vi "Inject Class Instances.vi"(8 "error in (no error)":errorcluster, 9 "Step in":refnum<class "CallVIStep.lvclass">, 10 "Execution in":refnum<data-value>, 11 "VI Refnum in":refnum<vi>) -> (0 "error out":errorcluster, 3 "VI Refnum out":refnum<vi>)   [LabVIEW 2015, in "CallVIStep.lvclass"]
uses:
  CallVIStep.lvclass
  Execution.lvclass
  Project.lvclass
  <vilib>/Utility/Data Type/NI_Data Type.lvlib
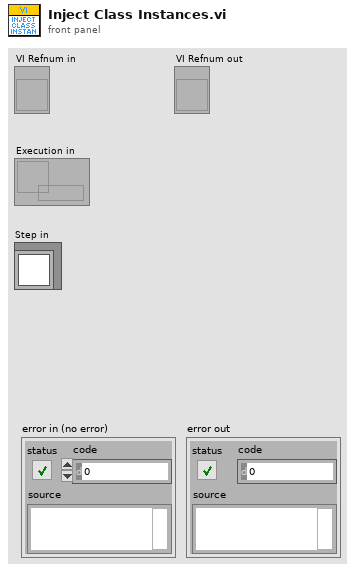
[diagram p1: front panel]
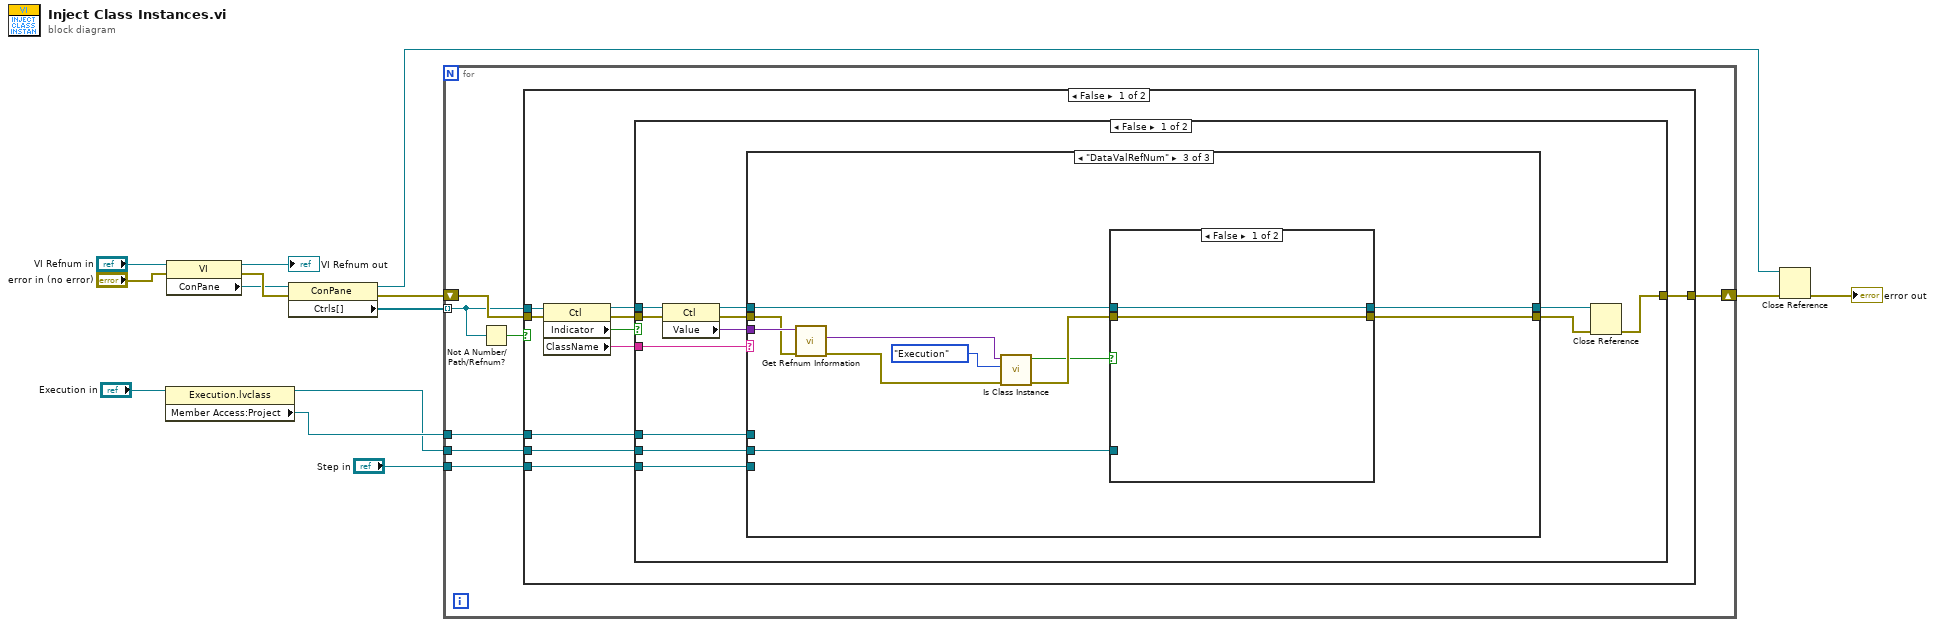
[diagram p0: block diagram]
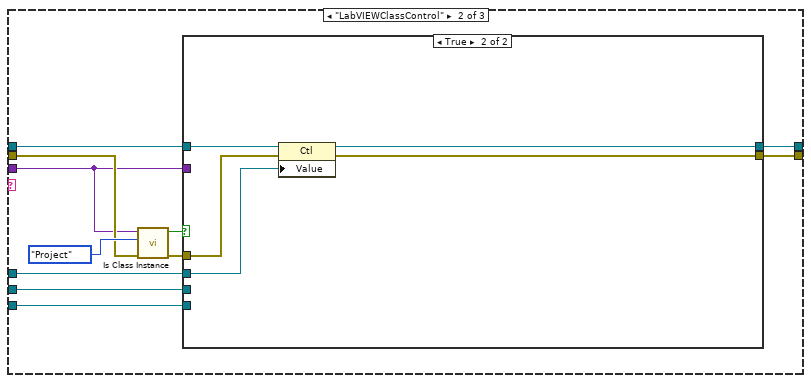
[diagram p3: hidden frame]
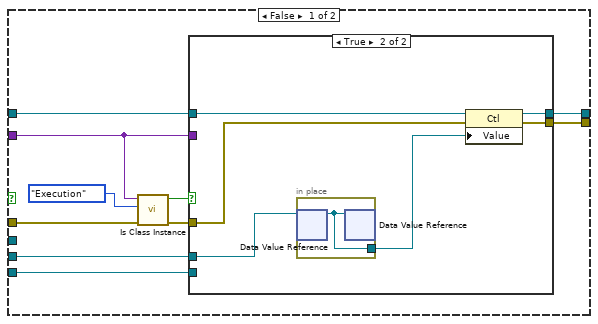
[diagram p4: hidden frame]
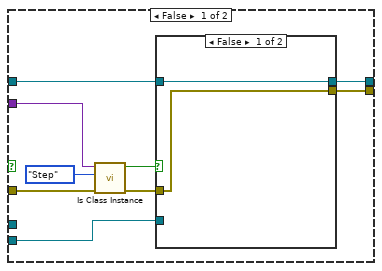
[diagram p5: hidden frame]
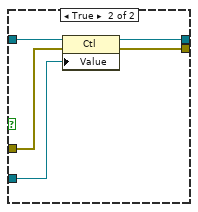
[diagram p6: hidden frame]
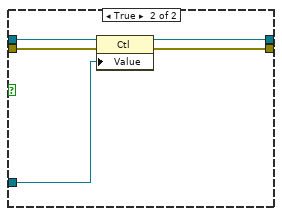
[diagram p7: hidden frame]
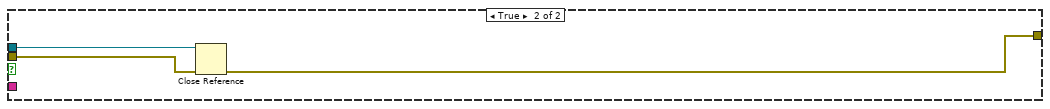
[diagram p8: hidden frame]
diagram:
  n1 = property class="Execution.lvclass"(reference="Execution in") -> (reference out=w1:refnum<data-value>, "Member Access:Project"=w2:refnum<class "Project.lvclass">)  [unwired: 1 in, 1 out]
  n2 = property class="VI"(reference="VI Refnum in", error in="error in (no error)") -> (reference out=→"VI Refnum out":refnum<vi>, error out=w13:errorcluster, "ConPane"=w11:refnum<vi>)
  n3 = property class="ConPane"(reference=w11, error in=w13) -> (reference out=w6:refnum<vi>, error out=w14:errorcluster, "Ctrls[]"=w12:refnum<vi>[])
  n4 = for {
    tunnel: w12 -> [w18] mode=indexing
    tunnel: w2 -> [w20]
    shift-right: [w19] -> w7
    shift-left: w14 -> [w21]
    tunnel: w1 -> [w16]
    tunnel: "Step in" -> [w15]
    n5 = Not A Number/Path/Refnum?(number/path/refnum=w18) -> (NaN/Path/Refnum?=w17:bool)
    n6 = case shown="False" w17 {
      tunnel: w21 -> [w31 w116]
      tunnel: w20 -> [w28 _]
      tunnel: [w27 w116] -> w19
      tunnel: w18 -> [w26 _]
      tunnel: w16 -> [w25 _]
      tunnel: w15 -> [w24 _]
      frame False {
        n7 = property class="Ctl"(reference=w26, error in=w31) -> (reference out=w30:refnum<vi>, error out=w29:errorcluster, "Indicator"=w23:bool, "ClassName"=w22:string)
        n8 = case shown="False" w23 {
          tunnel: w30 -> [w36 w115]
          tunnel: w29 -> [w35 w114]
          tunnel: w28 -> [w40 _]
          tunnel: [w41 w113] -> w27
          tunnel: w25 -> [w39 _]
          tunnel: w24 -> [w38 _]
          tunnel: w22 -> [w37 _]
          frame False {
            n9 = property class="Ctl"(reference=w36, error in=w35) -> (reference out=w34:refnum<vi>, error out=w33:errorcluster, "Value"=w32:variant)
            n10 = case shown="\"DataValRefNum\"" w37 {
              tunnel: w34 -> [w45 w48 w100]
              tunnel: w33 -> [w44 w47 w102]
              tunnel: [w45 w54 w96] -> w43
              tunnel: [w44 w53 w95] -> w42
              tunnel: w40 -> [_ w52 _]
              tunnel: w39 -> [_ w50 w97]
              tunnel: w38 -> [_ w49 _]
              tunnel: w32 -> [_ w46 w105]
              frame Default {
              }
              frame "LabVIEWClassControl" {
                n11 = call "Is Class Instance.vi"("error in (no error)"=w47, "Class Type"=enum16{"Project", "Execution", "Step"}."Project", "Control Value"=w46) -> ("error out"=w55:errorcluster, "Is Class Instance"=w56:bool)  [unwired: 5 in, 2 out]
                n12 = case shown="True" w56 {
                  tunnel: w48 -> [w63 w94]
                  tunnel: w55 -> [w65 w92]
                  tunnel: w52 -> [_ w93]
                  tunnel: [w60 w91] -> w54
                  tunnel: [w57 w90] -> w53
                  tunnel: w46 -> [w59 _]
                  tunnel: w50 -> [w62 _]
                  tunnel: w49 -> [w58 _]
                  frame False {
                    n13 = call "Is Class Instance.vi"("error in (no error)"=w65, "Class Type"=enum16{"Project", "Execution", "Step"}."Execution", "Control Value"=w59) -> ("error out"=w61:errorcluster, "Is Class Instance"=w64:bool)  [unwired: 5 in, 2 out]
                    n14 = case shown="True" w64 {
                      tunnel: w63 -> [w70 w88]
                      tunnel: w62 -> [_ w84]
                      tunnel: w61 -> [w75 w87]
                      tunnel: [w69 w86] -> w60
                      tunnel: w59 -> [w74 _]
                      tunnel: w58 -> [w68 _]
                      tunnel: [w67 w85] -> w57
                      frame False {
                        n15 = call "Is Class Instance.vi"("error in (no error)"=w75, "Class Type"=enum16{"Project", "Execution", "Step"}."Step", "Control Value"=w74) -> ("error out"=w71:errorcluster, "Is Class Instance"=w72:bool)  [unwired: 5 in, 2 out]
                        n16 = case shown="False" w72 {
                          tunnel: w71 -> [w76 w79]
                          tunnel: w70 -> [w77 w82]
                          tunnel: [w77 w81] -> w69
                          tunnel: w68 -> [_ w80]
                          tunnel: [w76 w78] -> w67
                          frame False {
                          }
                          frame True {
                            n17 = property class="Ctl"(reference=w82, error in=w79, "Value"=w80) -> (reference out=w81:refnum<vi>, error out=w78:errorcluster)
                          }
                        }
                      }
                      frame True {
                        n18 = in-place {
                          in-place-border: [w89] -> w83
                          n19 = in-place-dvr #1(w84) -> (w89:refnum<class "Execution.lvclass">)  [unwired: 1 out]
                          n20 = in-place-dvr #1(w89) -> ()  [unwired: 2 out]
                        }
                        n21 = property class="Ctl"(reference=w88, error in=w87, "Value"=w83) -> (reference out=w86:refnum<vi>, error out=w85:errorcluster)
                      }
                    }
                  }
                  frame True {
                    n22 = property class="Ctl"(reference=w94, error in=w92, "Value"=w93) -> (reference out=w91:refnum<vi>, error out=w90:errorcluster)
                  }
                }
              }
              frame "DataValRefNum" {
                n23 = call <vilib>:"Get Refnum Information.vi"("error in (no error)"=w102, "Variant"=w105) -> ("error out"=w101:errorcluster, "Strict Type"=w103:variant)  [unwired: 6 in, 2 out]
                n24 = call "Is Class Instance.vi"("error in (no error)"=w101, "Class Type"=enum16{"Project", "Execution", "Step"}."Execution", "Control Value"=w103) -> ("error out"=w99:errorcluster, "Is Class Instance"=w98:bool)  [unwired: 5 in, 2 out]
                n25 = case shown="False" w98 {
                  tunnel: w100 -> [w107 w112]
                  tunnel: w99 -> [w106 w111]
                  tunnel: w97 -> [_ w110]
                  tunnel: [w107 w109] -> w96
                  tunnel: [w106 w108] -> w95
                  frame False {
                  }
                  frame True {
                    n26 = property class="Ctl"(reference=w112, error in=w111, "Value"=w110) -> (reference out=w109:refnum<vi>, error out=w108:errorcluster)
                  }
                }
              }
            }
            n27 = Close Reference(reference=w43, error in (no error)=w42) -> (error out=w41:errorcluster)
          }
          frame True {
            n28 = Close Reference(reference=w115, error in (no error)=w114) -> (error out=w113:errorcluster)
          }
        }
      }
      frame True {
      }
    }
  }
  n29 = Close Reference(reference=w6, error in (no error)=w7) -> (error out=→"error out":errorcluster)
